vi "Write U8.vi"(7 "RegisterOffset":u32, 8 "error in":errorcluster, 9 "value in":u8, 10 "register name":string, 11 "session in":u32) -> (0 "error out":errorcluster, 3 "session out":u32)   [LabVIEW 2024, in "FPGA Register IO.lvlib"]
uses:
  FPGA Register IO.lvlib
  NiFpga.dll
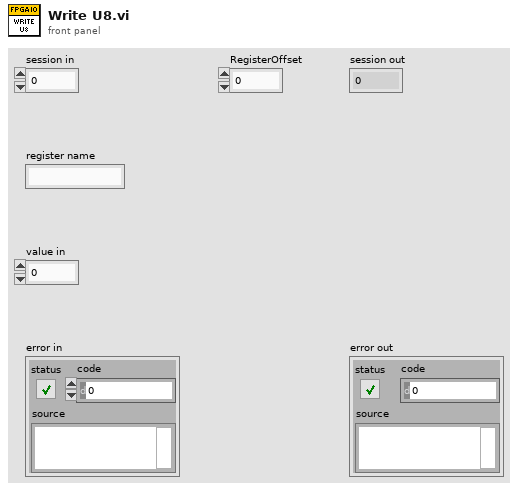
[diagram p1: front panel]
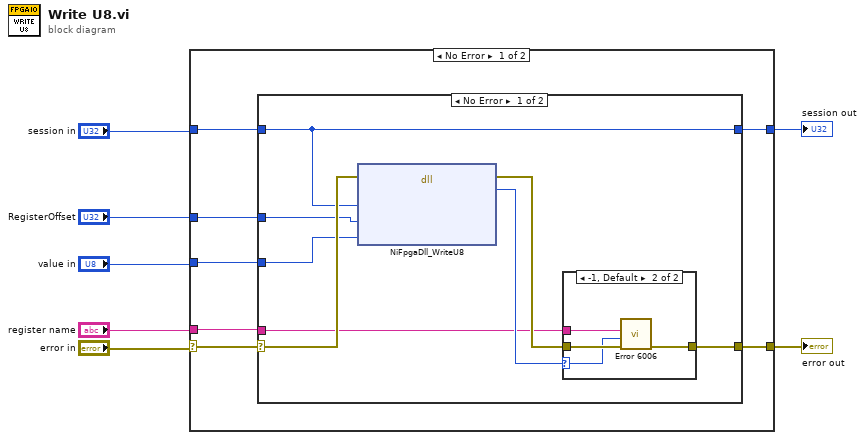
[diagram p0: block diagram]
diagram:
  n1 = case shown="No Error" "error in" {
    selector: "error in" -> [w9 w30]
    tunnel: "session in" -> [w10 w31]
    tunnel: [w14 w30] -> w6
    tunnel: [w13 w31] -> w5
    tunnel: "value in" -> [w12 _]
    tunnel: "register name" -> [w11 _]
    tunnel: "RegisterOffset" -> [w8 _]
    frame No Error {
      n2 = case shown="No Error" w9 {
        selector: w9 -> [w22 w29]
        tunnel: w10 -> [w21 w28]
        tunnel: [w19 w29] -> w14
        tunnel: [w21 w28] -> w13
        tunnel: w12 -> [w20 _]
        tunnel: w11 -> [w16 _]
        tunnel: w8 -> [w15 _]
        frame No Error {
          n3 = dll-call lib="NiFpga.*" fn="NiFpgaDll_WriteU8"(error in=w22, "session"=w21, "offset"=w15, "value"=w20) -> (error out=w18:errorcluster, "status"=w17:i32)  [unwired: 5 in, 1 out]
          n4 = case shown="-1, Default" w17 {
            selector: w17 -> [_ w25]
            tunnel: w18 -> [w23 w26]
            tunnel: [w23 w27] -> w19
            tunnel: w16 -> [_ w24]
            frame 0 {
            }
            frame -1, Default {
              n5 = call "Error 6006.vi"("error in (no error)"=w26, "rio status code"=w25, "register name"=w24) -> ("error out"=w27:errorcluster)  [unwired: 8 in]
            }
          }
        }
        frame Error {
        }
      }
    }
    frame Error {
    }
  }
  "error out" <- w6
  "session out" <- w5
